vi "Main_11A.vi"() -> ()   [LabVIEW 2024]
panel:
  in  "Example 2":string="125 17"
  in  "Use Puzzle":bool
  out "Answer 191690":u32
  in  "Puzzle":string="30 71441 3784 580926 2 8122942 0 291"
  in  "Example":string="0 1 10 99 999"
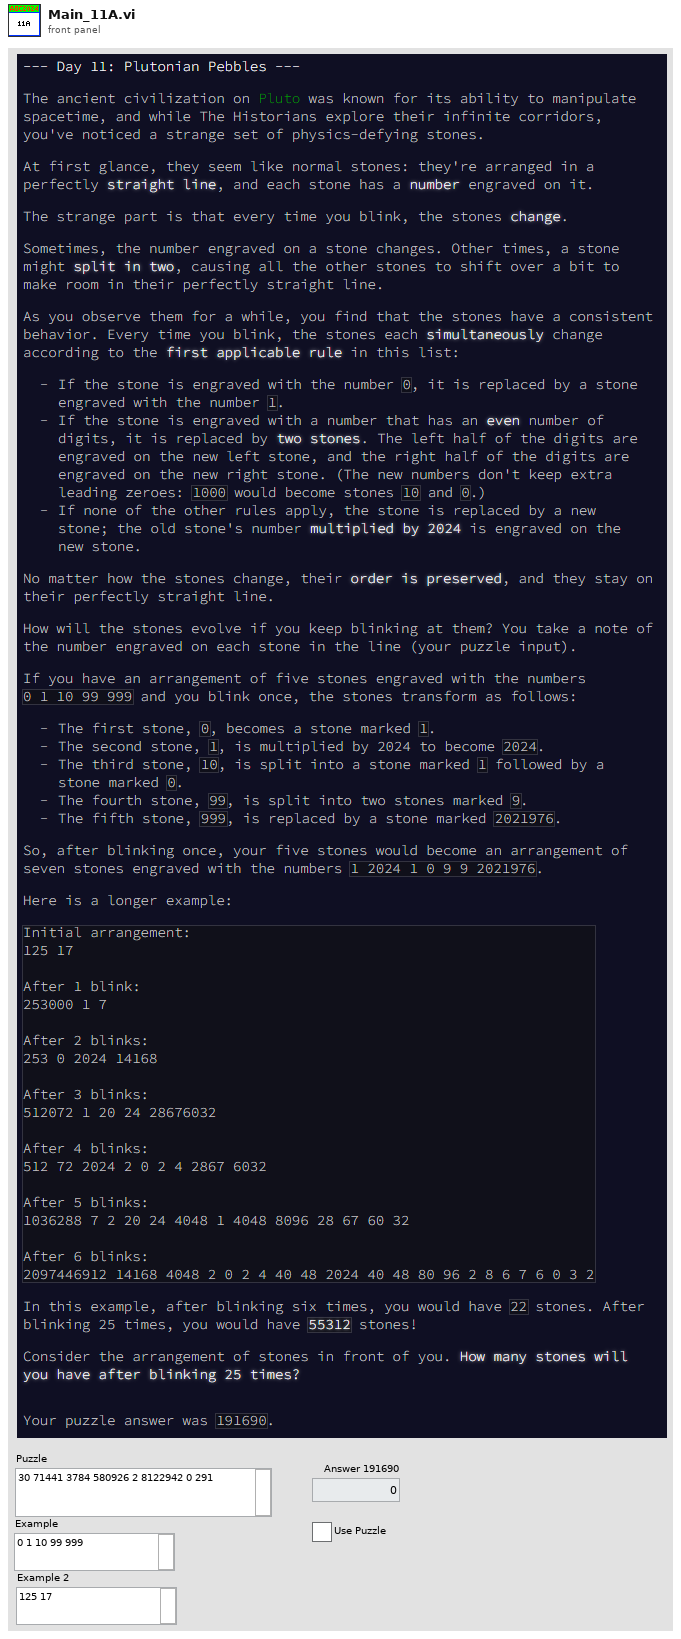
[diagram p1: front panel]
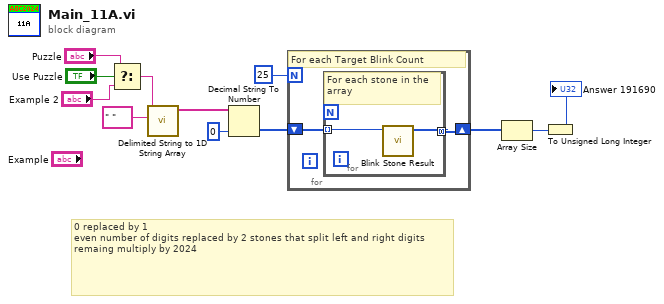
[diagram p0: block diagram]
diagram:
  # "0 replaced by 1\neven number of digits replaced by 2 stones that split left and right digits\nremaing multiply by 2024"
  n1 = Select(t="Puzzle", s="Use Puzzle", f="Example 2") -> (s? t:f=w10:string)
  n2 = call <vilib>:"Delimited String to 1D String Array.vi"("delimiter"=" " ("delimiter (Tab)"), "delimited string"=w10) -> ("string array"=w11:string[])  [unwired: 9 in]
  n3 = Decimal String To Number(string=w11, default (0L)=u64 0 ("default (0 I32)")) -> (number=w6:u64[])  [unwired: 1 in, 1 out]
  n4 = for {
    N: 25 -> [_]
    shift-right: [w14] -> w1
    shift-left: w6 -> [w13]
    # "For each Target Blink Count"
    n5 = for {
      tunnel: w13 -> [w16] mode=indexing
      tunnel: [w15] -> w14 mode=concatenating
      # "For each stone in the array"
      n6 = call "Blink Stone Result.vi"("String"=w16) -> ("Result Array"=w15:u64[])  [unwired: 9 in, 1 out]
    }
  }
  n7 = Array Size(array=w1) -> (size(s)=w3:i32)
  n8 = To Unsigned Long Integer(number=w3) -> (unsigned 32bit integer=→"Answer 191690":u32)
